vi "Cluster-UnbundleByName.vi"() -> ()   [LabVIEW 2019]
panel:
  in  "Cluster":T1 {"Slide 2" scale=0.0..10.0; "Slide 1" scale=0.0..10.0}
  out "Gauge":dbl(knob) scale=0.0..10.0
  # "LabVIEW Cluster Demonstration"
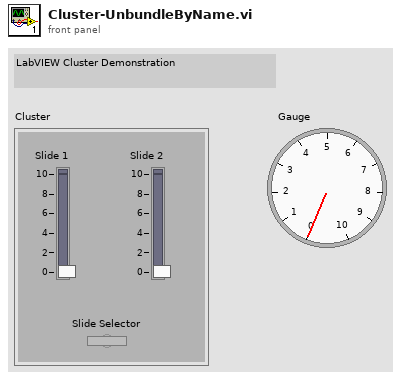
[diagram p1: front panel]
types:
  T1 = cluster{"Slide 1":dbl, "Slide 2":dbl, "Slide Selector":bool}
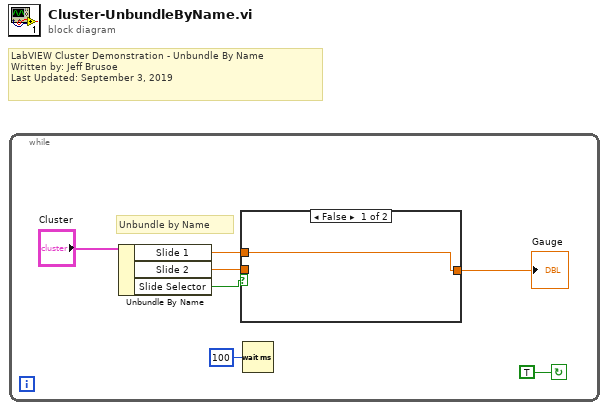
[diagram p0: block diagram]
diagram:
  # "LabVIEW Cluster Demonstration - Unbundle By Name\nWritten by: Jeff Brusoe\nLast Updated: September 3, 2019"
  n1 = while {
    stop <- TRUE continue-if-true
    # "Unbundle by Name"
    n2 = Unbundle By Name("Cluster") -> ("Slide 1"=w2:dbl, "Slide 2"=w3:dbl, "Slide Selector"=w5:bool)
    n3 = case shown="False" w5 {
      tunnel: [w8 w9] -> w4
      tunnel: w3 -> [_ w9]
      tunnel: w2 -> [w8 _]
      frame False {
      }
      frame True {
      }
    }
    "Gauge" <- w4
    n4 = Wait (ms)(milliseconds to wait=u32 100) -> ()  [unwired: 1 out]
  }
